vi "Register gRPC Methods.vi"(8 "error in (no error)":errorcluster, 11 "Template Server in":refnum<class "HVC2.lvclass">) -> (0 "error out":errorcluster, 3 "Template Server out":refnum<class "HVC2.lvclass">)   [LabVIEW 2019, in "HVC2.lvlib" / "HVC2.lvclass"]
uses:
  HVC2.lvclass
  typeDefs/Server Internal UEs.ctl
  typeDefs/Server Internal Message.ctl
  typeDefs/Server gRPC UEs.ctl
  gRPC lvSupport/Server API/typeDefs/gRPCId Cluster.ctl
  gRPC lvSupport/Server API/typeDefs/grpcId.ctl
  HVC2.lvclass/HVC2.ctl
  gRPC lvSupport/gprc-lvsupport.lvlib
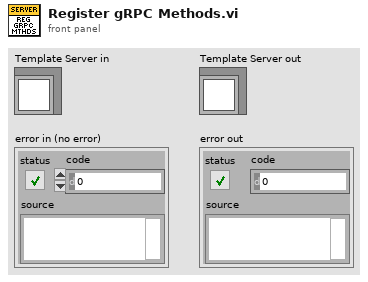
[diagram p1: front panel]
types:
  T1 = typedef "HVC2.lvlib/HVC2.lvclass/Server gRPC UEs.ctl" = cluster{"Invoke gRPC UE":refnum<user-event>, "Query gRPC UE":refnum<user-event>, "Register gRPC UE":refnum<user-event>, "ConfigureDMM gRPC UE":refnum<user-event>, "PerformDMMVoltageMeasurement gRPC UE":refnum<user-event>}
  T2 = typedef "HVC2.lvlib/HVC2.lvclass/Server Internal UEs.ctl" = cluster{"Invoke Internal UE":refnum<user-event>, "Query Internal UE":refnum<user-event>, "Register Internal UE":refnum<user-event>, "ConfigureDMM Internal UE":refnum<user-event>, "PerformDMMVoltageMeasurement Internal UE":refnum<user-event>}
  T3 = typedef "HVC2.lvlib/gprc-lvsupport.lvlib/grpcId.ctl" = u64
  T4 = typedef "HVC2.lvlib/HVC2.lvclass/Server Internal Message UE.ctl" = refnum<user-event>
  T5 = typedef "HVC2.lvlib/gprc-lvsupport.lvlib/gRPCId Cluster UE.ctl" = refnum<user-event>
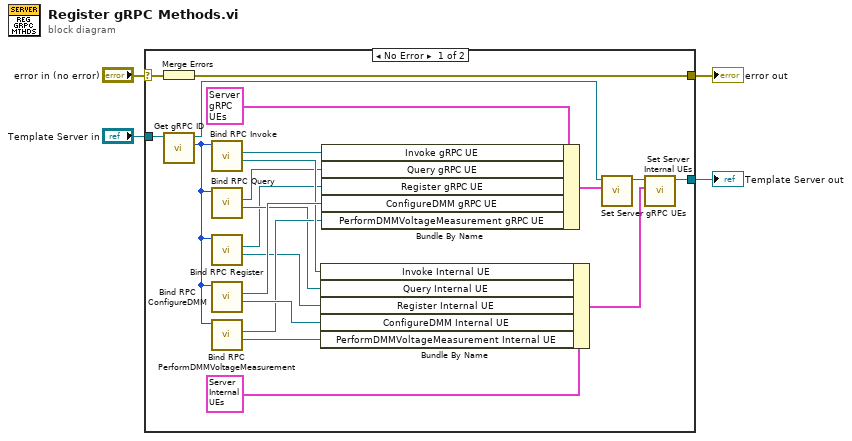
[diagram p0: block diagram]
diagram:
  n1 = case shown="No Error" "error in (no error)" {
    selector: "error in (no error)" -> [w16 w26]
    tunnel: "Template Server in" -> [w24 w27]
    tunnel: [w23 w26] -> w3
    tunnel: [w22 w27] -> w2
    frame No Error {
      n2 = Merge Errors(w16) -> (w23:errorcluster)
      n3 = call "Get gRPC ID.vi"("OOP Server in"=w24) -> ("gRPC ID"=w15:T3, "OOP Server out"=w25:refnum<class "HVC2.lvclass">)  [unwired: 9 in]
      n4 = call "Bind RPC Invoke.vi"("gRPCid server in"=w15) -> ("Invoke Internal UE"=w12:T4, "Invoke gRPC UE"=w11:T5)  [unwired: 7 in, 2 out]
      n5 = call "Bind RPC Query.vi"("gRPCid server in"=w15) -> ("Query Internal UE"=w8:T4, "Query gRPC UE"=w7:T5)  [unwired: 7 in, 2 out]
      n6 = call "Bind RPC Register.vi"("gRPCid server in"=w15) -> ("Register Internal UE"=w6:T4, "Register gRPC UE"=w5:T5)  [unwired: 7 in, 2 out]
      n7 = call "Bind RPC ConfigureDMM.vi"("gRPCid server in"=w15) -> ("ConfigureDMM Internal UE"=w14:T4, "ConfigureDMM gRPC UE"=w13:T5)  [unwired: 7 in, 2 out]
      n8 = call "Bind RPC PerformDMMVoltageMeasurement.vi"("gRPCid server in"=w15) -> ("PerformDMMVoltageMeasurement Internal UE"=w10:T4, "PerformDMMVoltageMeasurement gRPC UE"=w9:T5)  [unwired: 7 in, 2 out]
      n9 = Bundle By Name ("Bundle Internal UEs")(cluster=T2 {"Invoke Internal UE"=refnum, "Query Internal UE"=refnum, "Register Internal UE"=refnum, "ConfigureDMM Internal UE"=refnum, "PerformDMMVoltageMeasurement Internal UE"=refnum} ("Server Internal UEs"), "Invoke Internal UE"=w12, "Query Internal UE"=w8, "Register Internal UE"=w6, "ConfigureDMM Internal UE"=w14, "PerformDMMVoltageMeasurement Internal UE"=w10) -> (w21:T2)
      n10 = Bundle By Name ("Bundle gRPC UEs")(cluster=T1 {"Invoke gRPC UE"=refnum, "Query gRPC UE"=refnum, "Register gRPC UE"=refnum, "ConfigureDMM gRPC UE"=refnum, "PerformDMMVoltageMeasurement gRPC UE"=refnum} ("gRPC Server Method Events"), "Invoke gRPC UE"=w11, "Query gRPC UE"=w7, "Register gRPC UE"=w5, "ConfigureDMM gRPC UE"=w13, "PerformDMMVoltageMeasurement gRPC UE"=w9) -> (w18:T1)
      n11 = call "Set Server gRPC UEs.vi"("Server gRPC UEs"=w18, "OOP Server in"=w25) -> ("OOP Server out"=w19:refnum<class "HVC2.lvclass">)  [unwired: 9 in]
      n12 = call "Set Server Internal UEs.vi"("Server Internal UEs"=w21, "OOP Server in"=w19) -> ("OOP Server out"=w22:refnum<class "HVC2.lvclass">)  [unwired: 9 in]
    }
    frame Error {
    }
  }
  "error out" <- w3
  "Template Server out" <- w2
